vi "Teleop.vi"(10 "Match Info":T1={"Autonomous Elapsed Seconds"=0.0, "TeleOp Elapsed Seconds"=0.0, "Disabled Elapsed Seconds"=0.0, "Visited Autonomous"=FALSE, "Visited TeleOp"=FALSE, "Visited Disabled"=FALSE, "Autonomous Settings"={"Autonomous Style"=enum."Independent", "VI Refnum"=refnum}}, 11 "Call Context":T2) -> ()   [LabVIEW 2019]
doc: "This VI is called for each TeleOp packet received from the DS where the robot is not disabled. It is often used to read from the joysticks and update I/O or to update setpoints for timed control loops. It should complete and return within 20 milliseconds or it may miss DS packets."
uses:
  <vilib>/Rock Robotics/WPI/DriverStation/WPI_DriverStationDerivedRobotMode.ctl
  <vilib>/Rock Robotics/WPI/DriverStation/WPI_DriverStationMatch Info.ctl
  <vilib>/Rock Robotics/WPI/ThirdParty/REV Robotics/SPARK MAX/Typedef/Spark MAX Control Type.ctl
  <vilib>/Rock Robotics/WPI/Solenoid/WPI_SolenoidValue.ctl
  <vilib>/Rock Robotics/WPI/Utilities/WPI_GetSetVariantRefNum.vi
  <vilib>/Rock Robotics/Network Tables/NT Write Number.vi
  <vilib>/Rock Robotics/WPI/Solenoid/WPI_SolenoidSetEnum.vi
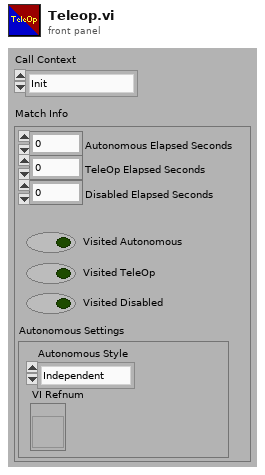
[diagram p1: front panel]
types:
  T1 = typedef "WPI_DriverStationMatch Info.ctl" = cluster{"Autonomous Elapsed Seconds":dbl, "TeleOp Elapsed Seconds":dbl, "Disabled Elapsed Seconds":dbl, "Visited Autonomous":bool, "Visited TeleOp":bool, "Visited Disabled":bool, "Autonomous Settings":cluster{"Autonomous Style":enum16{"Iterative", "Independent"}, "VI Refnum":refnum<vi>}}
  T2 = typedef "WPI_DriverStationDerivedRobotMode.ctl" = enum16{"Init", "Execute", "Stop"}
  T3 = typedef "WPI_SolenoidValue.ctl" = enum16{"Off", "On", "Forward", "Reverse"}
  T4 = typedef "Spark MAX Control Type.ctl" = enum16{"Percent VBus", "Voltage", "Velocity", "Position", "Smart Motion", "Current", "Smart Velocity"}
  T5 = typedef "WPI_JoystickDevRef.ctl" = cluster{"Device":T6}
  T6 = typedef "WPI_JoystickDeviceEnum.ctl" = enum16{"USB 0", "USB 1", "USB 2", "USB 3", "USB 4", "USB 5"}
  T7 = cluster{"POVs[0]":i16, "POVs[1]":i16, "POVs[2]":i16, "POVs[3]":i16, "POVs[4]":i16, "POVs[5]":i16, "POVs[6]":i16, "POVs[7]":i16, "POVs[8]":i16}
  T8 = cluster{"Axes[0]":dbl, "Axes[1]":dbl, "Axes[2]":dbl, "Axes[3]":dbl, "Axes[4]":dbl, "Axes[5]":dbl, "Axes[6]":dbl, "Axes[7]":dbl, "Axes[8]":dbl}
  T9 = cluster{"Buttons[0]":bool, "Buttons[1]":bool, "Buttons[2]":bool, "Buttons[3]":bool, "Buttons[4]":bool, "Buttons[5]":bool, "Buttons[6]":bool, "Buttons[7]":bool, "Buttons[8]":bool}
  T10 = typedef "WPI_MotorControlDeviceRef.ctl" = cluster{"DeviceStatus":errorcluster, "Type":T11, "PWM":cluster{"PWM Channel":T12, "DeadBand":T13}, "CAN":cluster{"Device Number":u8, "SetOutput VI Ref":variant, "GetOutput VI Ref":variant, "Enable VI Ref":variant, "Disable VI Ref":variant, "Data":variant}, "Invert":bool, "DIO PWM":cluster{"PWM \"Enable\" Channel":T12, "DIOChannel":T14, "PWM Rate":dbl}}
  T11 = typedef "WPI_MotorControlType.ctl" = enum16{"PWM", "CAN", "DIO PWM"}
  T12 = typedef "FPGA_DIOPWMChannel.ctl" = enum8{"PWM 0", "PWM 1", "PWM 2", "PWM 3", "PWM 4", "PWM 5", "PWM 6", "PWM 7", "PWM 8", "PWM 9", "PWM MXP 0", "PWM MXP 1", "PWM MXP 2", "PWM MXP 3", "PWM MXP 4", "PWM MXP 5", "PWM MXP 6", "PWM MXP 7", "PWM MXP 8", "PWM MXP 9", "Invalid"}
  T13 = typedef "WPI_PWMDeadband.ctl" = cluster{"Name":string, "maxPositivePwm":i32, "minPositivePwm":i32, "centerPwm":i32, "maxNegativePwm":i32, "minNegativePwm":i32, "angularRange":u16}
  T14 = typedef "FPGA_DIOChannel.ctl" = enum8{"DIO 0", "DIO 1", "DIO 2", "DIO 3", "DIO 4", "DIO 5", "DIO 6", "DIO 7", "DIO 8", "DIO 9", "DIO MXP 0", "DIO MXP 1", "DIO MXP 2", "DIO MXP 3", "DIO MXP 4", "DIO MXP 5", "DIO MXP 6", "DIO MXP 7", "DIO MXP 8", "DIO MXP 9", "DIO MXP 10", "DIO MXP 11", "DIO MXP 12", "DIO MXP 13", "DIO MXP 14", "DIO MXP 15", "SPI Port CS1", "SPI Port CS2", "SPI Port CS3", "SPI Port MISO", "SPI Port MOSI", "Invalid"}
  T15 = typedef "WPI_SolenoidDevRef.ctl" = cluster{"DevStatus":errorcluster, "Pneumatics Control Module":u8, "Forward Solenoid Channel":T16, "Reverse Solenoid Channel":T16}
  T16 = typedef "WPI_SolenoidChannel.ctl" = enum8{"Solenoid 0", "Solenoid 1", "Solenoid 2", "Solenoid 3", "Solenoid 4", "Solenoid 5", "Solenoid 6", "Solenoid 7", "Invalid"}
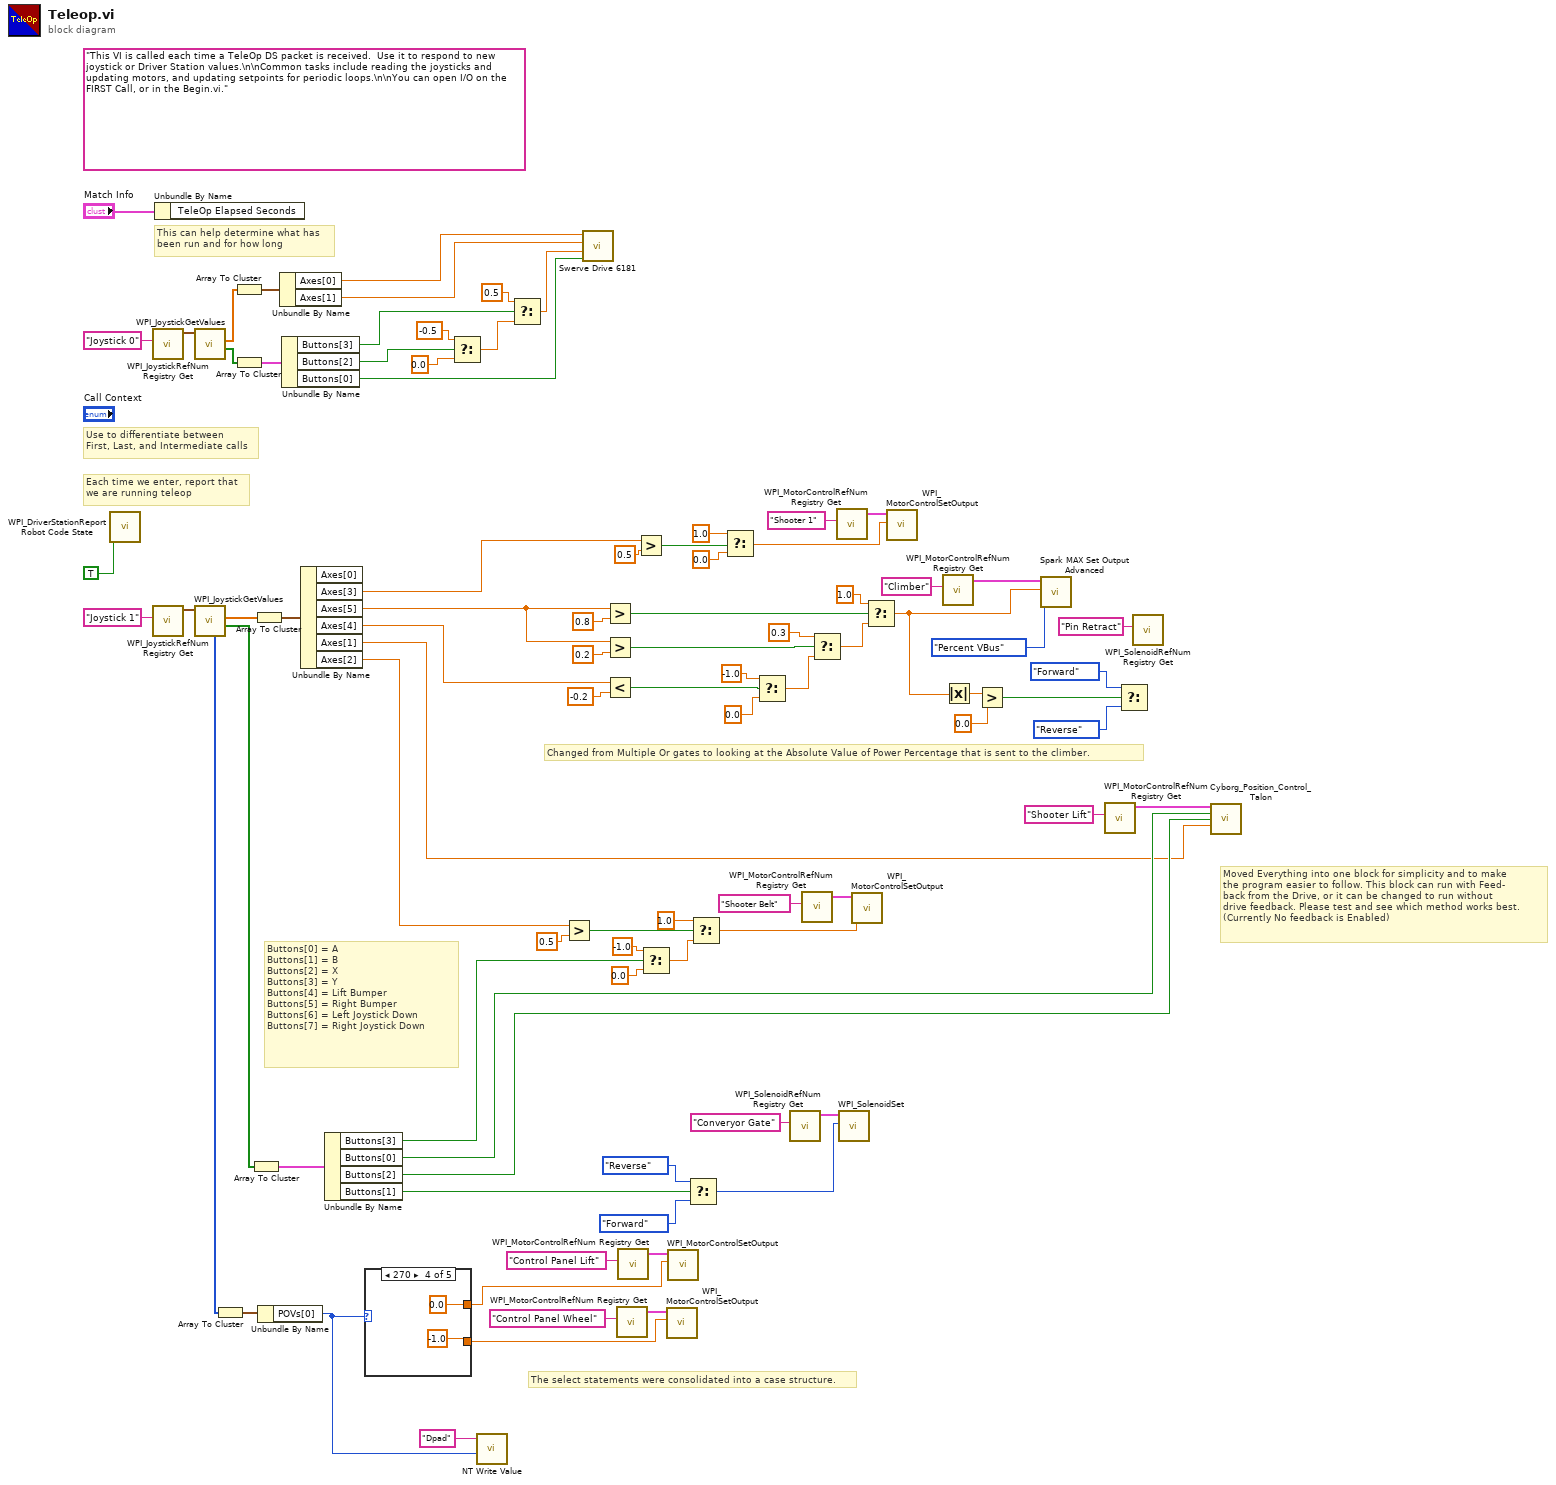
[diagram p0: block diagram]
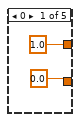
[diagram p2: hidden frame]
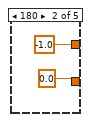
[diagram p3: hidden frame]
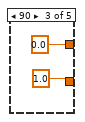
[diagram p4: hidden frame]
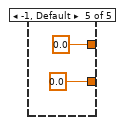
[diagram p5: hidden frame]
diagram:
  (unwired) "This VI is called each time a TeleOp DS packet is received.  Use it to respond to new joystick or Driver Station values.\n\nCommon tasks include reading the joysticks and updating motors, and updating setpoints for periodic loops.\n\nYou can open I/O on the FIRST Call, or in the Begin.vi."
  # "The select statements were consolidated into a case structure."
  # "Moved Everything into one block for simplicity and to make \nthe program easier to follow. This block can run with Feed-\nback from the Drive, or it can be changed to run without \ndrive feedback. Please test and see which method works best.\n(Currently No feedback is Enabled)"
  # "Changed from Multiple Or gates to looking at the Absolute Value of Power Percentage that is sent to the climber."
  # "Buttons[0] = A\nButtons[1] = B\nButtons[2] = X\nButtons[3] = Y\nButtons[4] = Lift Bumper\nButtons[5] = Right Bumper\nButtons[6] = Left Joystick Down\nButtons[7] = Right Joystick Down"
  # "Each time we enter, report that\nwe are running teleop"
  # "Use to differentiate between\nFirst, Last, and Intermediate calls"
  # "This can help determine what has\nbeen run and for how long"
  n1 = call <vilib>:"WPI_DriverStationReport Robot Code State.vi"("TeleOp"=TRUE ("Autonomous")) -> ()  [unwired: 10 in, 1 out]
  n2 = call <vilib>:"WPI_JoystickRefNum Registry Get.vi"("refnum name"="Joystick 0") -> ("JoystickDevRef"=w86:T5)  [unwired: 1 in, 9 out]
  n3 = call <vilib>:"WPI_JoystickRefNum Registry Get.vi"("refnum name"="Joystick 1") -> ("JoystickDevRef"=w66:T5)  [unwired: 1 in, 9 out]
  n4 = Unbundle By Name("Match Info") -> ()  [unwired: 1 out]
  n5 = call <vilib>:"WPI_JoystickGetValues.vi"("JoystickDevRef"=w86) -> ("Buttons"=w81:bool[], "Axes"=w84:dbl[])  [unwired: 6 in, 3 out]
  n6 = call <vilib>:"WPI_JoystickGetValues.vi"("JoystickDevRef"=w66) -> ("Buttons"=w70:bool[], "Axes"=w67:dbl[], "POVs"=w36:i16[])  [unwired: 6 in, 2 out]
  n7 = Array To Cluster(array=w36) -> (cluster=w37:T7)
  n8 = Array To Cluster(array=w84) -> (cluster=w83:T8)
  n9 = Array To Cluster(array=w81) -> (cluster=w82:T9)
  n10 = Array To Cluster(array=w70) -> (cluster=w69:T9)
  n11 = Array To Cluster(array=w67) -> (cluster=w68:T8)
  n12 = Unbundle By Name(w37) -> ("POVs[0]"=w15:i16)
  n13 = Unbundle By Name(w83) -> ("Axes[0]"=w74:dbl, "Axes[1]"=w73:dbl)
  n14 = Unbundle By Name(w82) -> ("Buttons[3]"=w76:bool, "Buttons[2]"=w75:bool, "Buttons[0]"=w71:bool)
  n15 = Unbundle By Name(w68) -> ("Axes[3]"=w55:dbl, "Axes[5]"=w7:dbl, "Axes[4]"=w6:dbl, "Axes[1]"=w8:dbl, "Axes[2]"=w1:dbl)  [unwired: 1 out]
  n16 = Unbundle By Name(w69) -> ("Buttons[3]"=w9:bool, "Buttons[0]"=w11:bool, "Buttons[2]"=w10:bool, "Buttons[1]"=w30:bool)
  n17 = case shown="270" w15 {
    tunnel: [1.0 ("t") -1.0 ("t") 0.0 ("t") 0.0 ("t") 0.0 ("t")] -> w14
    tunnel: [0.0 ("f") 0.0 ("f") 1.0 ("f") -1.0 ("f") 0.0 ("f")] -> w13
    frame 0 {
    }
    frame 180 {
    }
    frame 90 {
    }
    frame 270 {
    }
    frame -1, Default {
    }
  }
  n18 = Select(t=-0.5, s=w75, f=0.0) -> (s? t:f=w80:dbl)
  n19 = call-poly <vilib>:"NT Write Value.vi"("Numeric"=w15, "Name"="Dpad") -> ()  [unwired: 9 in, 1 out]
  n20 = Select(t=0.5, s=w76, f=w80) -> (s? t:f=w72:dbl)
  n21 = Greater?(x=w1, y=0.5) -> (0:w59:bool)
  n22 = call "Swerve Drive 6181.vi"("X"=w74, "Y"=w73, "Z"=w72, "Robot-Centric"=w71) -> ()  [unwired: 2 in, 1 out]
  n23 = Greater?(x=w7, y=0.8) -> (0:w16:bool)
  n24 = Greater?(x=w7, y=0.2) -> (0:w17:bool)
  n25 = Less?(x=w6, y=-0.2) -> (x < y?=w18:bool)
  n26 = call <vilib>:"WPI_MotorControlRefNum Registry Get.vi"("refnum name"="Control Panel Wheel") -> ("MotorControlDevRef"=w19:T10)  [unwired: 9 in, 1 out]
  n27 = call <vilib>:"WPI_MotorControlRefNum Registry Get.vi"("refnum name"="Control Panel Lift") -> ("MotorControlDevRef"=w21:T10)  [unwired: 9 in, 1 out]
  n28 = Greater?(x=w55, y=0.5) -> (0:w52:bool)
  n29 = Select(t=-1.0, s=w9, f=0.0) -> (s? t:f=w25:dbl)
  n30 = call <vilib>:"WPI_MotorControlSetOutput.vi"("Output"=w13, "MotorControlDevRef"=w19) -> ()  [unwired: 7 in, 3 out]
  n31 = call <vilib>:"WPI_MotorControlSetOutput.vi"("Output"=w14, "MotorControlDevRef"=w21) -> ()  [unwired: 7 in, 3 out]
  n32 = Select(t=WPI_SolenoidValue."Reverse" ("Value"), s=w30, f=WPI_SolenoidValue."Forward" ("Value")) -> (s? t:f=w29:T3)
  n33 = Select(t=1.0, s=w59, f=w25) -> (s? t:f=w60:dbl)
  n34 = Select(t=1.0, s=w52, f=0.0) -> (s? t:f=w51:dbl)
  n35 = Select(t=-1.0, s=w18, f=0.0) -> (s? t:f=w42:dbl)
  n36 = call <vilib>:"WPI_SolenoidRefNum Registry Get.vi"("refnum name"="Converyor Gate") -> ("SolenoidDevRef"=w34:T15)  [unwired: 9 in, 1 out]
  n37 = call <vilib>:"WPI_MotorControlRefNum Registry Get.vi"("refnum name"="Shooter Belt") -> ("MotorControlDevRef"=w61:T10)  [unwired: 9 in, 1 out]
  n38 = Select(t=0.3, s=w17, f=w42) -> (s? t:f=w46:dbl)
  n39 = call <vilib>:"WPI_MotorControlRefNum Registry Get.vi"("refnum name"="Shooter 1") -> ("MotorControlDevRef"=w53:T10)  [unwired: 9 in, 1 out]
  n40 = call-poly <vilib>:"WPI_SolenoidSet.vi"("Value"=w29, "SolenoidDevRef"=w34) -> ()  [unwired: 8 in, 2 out]
  n41 = call <vilib>:"WPI_MotorControlSetOutput.vi"("Output"=w60, "MotorControlDevRef"=w61) -> ()  [unwired: 7 in, 3 out]
  n42 = Select(t=1.0, s=w16, f=w46) -> (s? t:f=w3:dbl)
  n43 = call <vilib>:"WPI_MotorControlSetOutput.vi"("Output"=w51, "MotorControlDevRef"=w53) -> ()  [unwired: 7 in, 3 out]
  n44 = call <vilib>:"WPI_MotorControlRefNum Registry Get.vi"("refnum name"="Climber") -> ("MotorControlDevRef"=w39:T10)  [unwired: 9 in, 1 out]
  n45 = Absolute Value(x=w3) -> (abs(x)=w5:dbl)
  n46 = Greater?(x=w5, y=0.0) -> (0:w2:bool)
  n47 = call <vilib>:"Spark MAX Set Output Advanced.vi"("Control Mode"=Spark_MAX_Control_Type."Percent VBus", "Setpoint"=w3, "MotorControlDevRef"=w39) -> ()  [unwired: 7 in, 2 out]
  n48 = call <vilib>:"WPI_MotorControlRefNum Registry Get.vi"("refnum name"="Shooter Lift") -> ("MotorControlDevRef"=w12:T10)  [unwired: 9 in, 1 out]
  n49 = Select(t=WPI_SolenoidValue."Forward" ("Value"), s=w2, f=WPI_SolenoidValue."Reverse" ("Value")) -> ()  [unwired: 1 out]
  n50 = call <vilib>:"WPI_SolenoidRefNum Registry Get.vi"("refnum name"="Pin Retract") -> ()  [unwired: 9 in, 2 out]
  n51 = call "Cyborg_Position_Control_Talon.vi"("PhoenixMotorControlDevRef"=w12, "Upper"=w11, "Lower"=w10, "Jog Input"=w8) -> ()  [unwired: 12 in]
